vi "WriteIdentifierTest.vi"(6 "serial_number":string, 7 "part_number":string, 8 "error in (no error)":errorcluster, 9 "revision":string, 10 "method":string, 11 "Sequence Context In":refnum<k7>) -> (0 "error out":errorcluster, 2 "status":string)   [LabVIEW 2021]
uses:
  <vilib>/addons/TestStand/_TSUtility.llb/TestStand - Get Property Value (String).vi
  <vilib>/NI/JSON Support for LabVIEW/JSON Value/New JSON Value/New JSON ({String}).vi
  <vilib>/NI/JSON Support for LabVIEW/JSON Value/Object/Insert Value/Insert Value (String).vi
  <vilib>/NI/NI JSONRPC Server Framework/Classes/Client/Format Client Request (Auto-Increment).vi
  <vilib>/NI/NI JSONRPC Server Framework/Classes/Client/JSONRPC Client.lvclass
  <vilib>/NI/JSON Support for LabVIEW/JSON Value/JSON Value.lvclass
panel:
  out "description":string
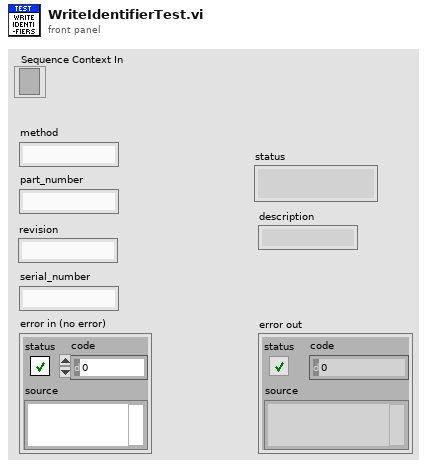
[diagram p1: front panel]
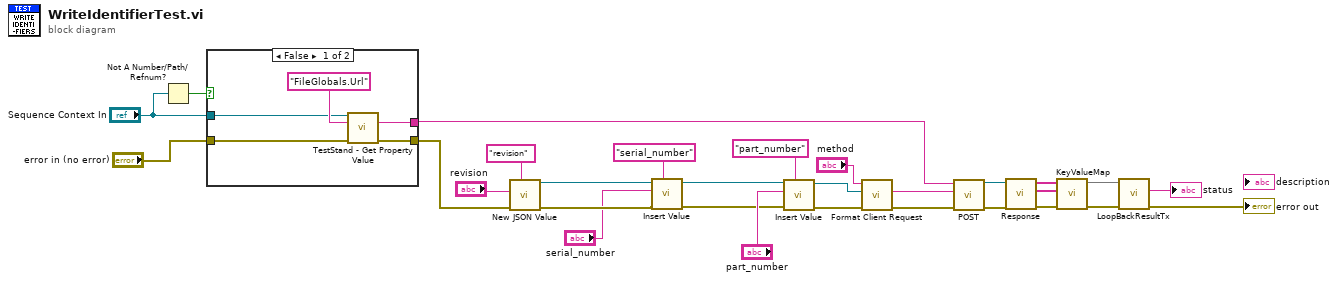
[diagram p0: block diagram]
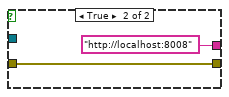
[diagram p2: hidden frame]
diagram:
  n1 = Not A Number/Path/Refnum?(number/path/refnum="Sequence Context In") -> (NaN/Path/Refnum?=w9:bool)
  n2 = case shown="False" w9 {
    tunnel: [w33 "http://localhost:8008" ("Value")] -> w29
    tunnel: [w32 w35] -> w16
    tunnel: "error in (no error)" -> [w31 w35]
    tunnel: "Sequence Context In" -> [w30 _]
    frame False {
      n3 = call-poly <vilib>:"TestStand - Get Property Value.vi"("Sequence Context In"=w30, "Lookup String"="FileGlobals.Url", "error in (no error)"=w31) -> ("Value"=w33:string, "error out"=w32:errorcluster)  [unwired: 10 in, 1 out]
    }
    frame True {
    }
  }
  n4 = call-poly <vilib>:"New JSON Value.vi"("key"="revision", "error in (no error)"=w16, "value"="revision") -> ("error out"=w7:errorcluster, "JSON Value out"=w5:refnum<class "JSON Value.lvclass">)  [unwired: 7 in]
  n5 = call-poly <vilib>:"Insert Value.vi"("key"="serial_number", "error in (no error)"=w7, "value"="serial_number", "JSON Value in"=w5) -> ("error out"=w6:errorcluster, "JSON Value out"=w4:refnum<class "JSON Value.lvclass">)  [unwired: 5 in, 1 out]
  n6 = call-poly <vilib>:"Insert Value.vi"("key"="part_number", "error in (no error)"=w6, "value"="part_number", "JSON Value in"=w4) -> ("error out"=w13:errorcluster, "JSON Value out"=w12:refnum<class "JSON Value.lvclass">)  [unwired: 5 in, 1 out]
  n7 = call-poly <vilib>:"Format Client Request.vi"("error in (no error)"=w13, "JSON Value in"=w12, "method"="method") -> ("error out"=w21:errorcluster, "Request String"=w15:string)  [unwired: 7 in]
  n8 = call "POST.vi"("error in (no error)"=w21, "Request String"=w15, "url"=w29) -> ("error out"=w22:errorcluster, "JSON Value out"=w23:refnum<class "JSON Value.lvclass">)  [unwired: 7 in]
  n9 = call "Response.vi"("error in (no error)"=w22, "JSON Value in"=w23) -> ("error out"=w24:errorcluster, "values"=w26:string[], "keys"=w25:string[])  [unwired: 7 in]
  n10 = call "KeyValueMap.vi"("error in"=w24, "values"=w26, "keys"=w25) -> ("error out"=w19:errorcluster, "map out"=w20:map{string, string})  [unwired: 7 in]
  n11 = call "LoopBackResultTx.vi"("error in (no error)"=w19, "map"=w20) -> ("error out"=→"error out":errorcluster, "status"=→"status":string)  [unwired: 8 in]
